vi "Write Poll List.vi"(8 "error in (no error)":errorcluster, 10 "Poll List":T1[](array[typedef]), 11 "MB PLC Client in":refnum<class "MB PLC Client.lvclass">) -> (0 "error out":errorcluster, 3 "MB PLC Client out":refnum<class "MB PLC Client.lvclass">)   [LabVIEW 2018, in "MB PLC Client.lvlib" / "MB PLC Client.lvclass"]
uses:
  MB PLC Client.lvclass
  Types/MB Ref Range_Cluster.ctl
  MB PLC Client.lvclass/MB PLC Client.ctl
  MB PLC Client.lvlib
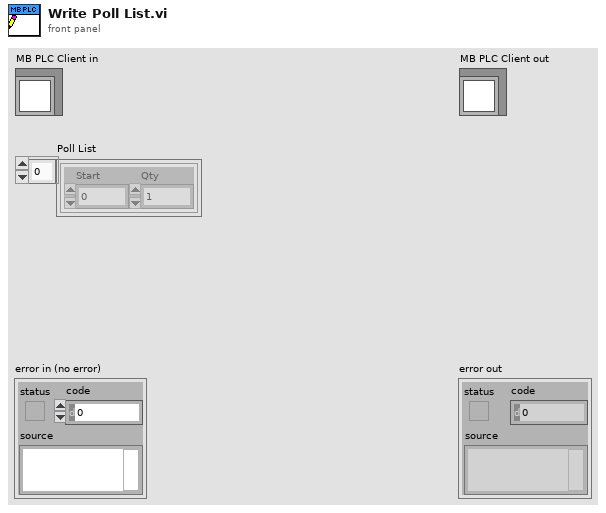
[diagram p1: front panel]
types:
  T1 = typedef "MB PLC Client.lvlib/MB Ref Range_Cluster.ctl" = cluster{"Start":u32, "Qty":u16}
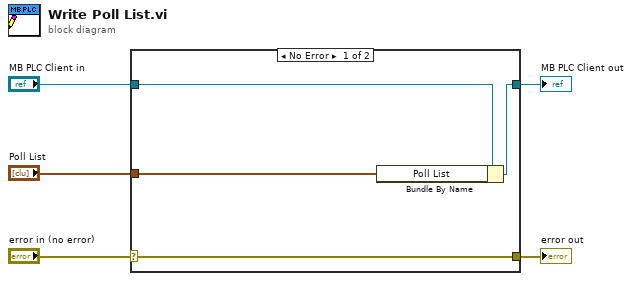
[diagram p0: block diagram]
diagram:
  n1 = case shown="No Error" "error in (no error)" {
    selector: "error in (no error)" -> [w9 w10]
    tunnel: [w9 w10] -> w4
    tunnel: [w7 w11] -> w2
    tunnel: "MB PLC Client in" -> [w8 w11]
    tunnel: "Poll List" -> [w6 _]
    frame No Error {
      n2 = Bundle By Name(cluster=w8, "Poll List"=w6) -> (w7:refnum<class "MB PLC Client.lvclass">)
    }
    frame Error {
    }
  }
  "error out" <- w4
  "MB PLC Client out" <- w2
